vi "Perform Memory Polynomial.vi"(0 "RFmx Instrument Handle In":refnum<k21>, 1 "Selector String":string, 5 "RFSG Instrument Handle In":refnum<k15>, 7 "Reference Waveform":T2={"Name"="Wfm", "Data"=refnum, "Signal Bandwidth (Hz)"=0.0, "PAPR (dB)"=0.0, "Burst Length (s)"=0.0, "Sample Rate"=0.0, "Burst Start Locations"=[], "Burst Stop Locations"=[], "Idle Duration Present?"=FALSE, "Runtime Scaling"=0.0, "Script"=""} {"Runtime Scaling" format="%#_6p"; "Sample Rate" format="%#_6p"; "Burst Length (s)" format="%#_6p"; "PAPR (dB)" format="%.2f"; "Signal Bandwidth (Hz)" format="%#_6p"}, 9 "Memory Polynomial Configuration":T4={"Correction Type"=0, "Number of Iterations"=3, " Order"=3, " Depth"=2, "Lead Order"=2, "Lag Order"=2, "Lead Memory Depth"=2, "Lag Memory Depth"=2, "Maximum Lead"=2, "Maximum Lag"=2} {"Number of Iterations" min=1; "Correction Type" items=["Magnitude and Phase", "Magnitude Only", "Phase Only"]}, 11 "error in (no error)":errorcluster) -> (4 "RFmx Instrument Handle Out":refnum<k21> caption="Instrument Handle Out", 6 "RFSG Instrument Handle Out":refnum<k15>, 8 "Memory Polynomial Results":T1={"Predistorted Waveform"={"Name"="Wfm", "Data"=refnum, "Signal Bandwidth (Hz)"=0.0, "PAPR (dB)"=0.0, "Burst Length (s)"=0.0, "Sample Rate"=0.0, "Burst Start Locations"=[], "Burst Stop Locations"=[], "Idle Duration Present?"=FALSE, "Runtime Scaling"=0.0, "Script"=""}, "Polynomial"=[], "Power Results"={"Waveform Power Offset (dB)"=-1.0, "Waveform True PAPR (dB)"=0.0, "Training Power (dBm)"=0.0}} {"Power Results"."Training Power (dBm)" format="%.2f"; "Power Results"."Waveform True PAPR (dB)" format="%.2f"; "Power Results"."Waveform Power Offset (dB)" format="%.2f"; "Predistorted Waveform"."Runtime Scaling" format="%#_6p"; "Predistorted Waveform"."Sample Rate" format="%#_6p"; "Predistorted Waveform"."Burst Length (s)" format="%#_6p"; "Predistorted Waveform"."PAPR (dB)" format="%.2f"; "Predistorted Waveform"."Signal Bandwidth (Hz)" format="%#_6p"; "Polynomial" format="%.2f"}, 15 "error out":errorcluster)   [LabVIEW 2019, in "RFmxDPD.lvlib"]
doc: "Acquires the incoming signal, trains the DPD model, applies the memory polynomial to the reference waveform, and downloads the predistorted waveform to the generator. If generation is in progress when this function is called, generation will resume with the predistorted waveform."
uses:
  RFmxDPD.lvlib
  Common/Waveform.ctl
  Typedefs/Memory Polynomial Configuration.ctl
  Typedefs/Memory Polynomial Results.ctl
  Typedefs/Power Results.ctl
  <vilib>/RFmx/SpecAn/mx/RFmxSpecAn.llb/RFmxSpecAn DPD Fetch DPD Polynomial.vi
  SG/SG.lvlib
  Common/Common.lvlib
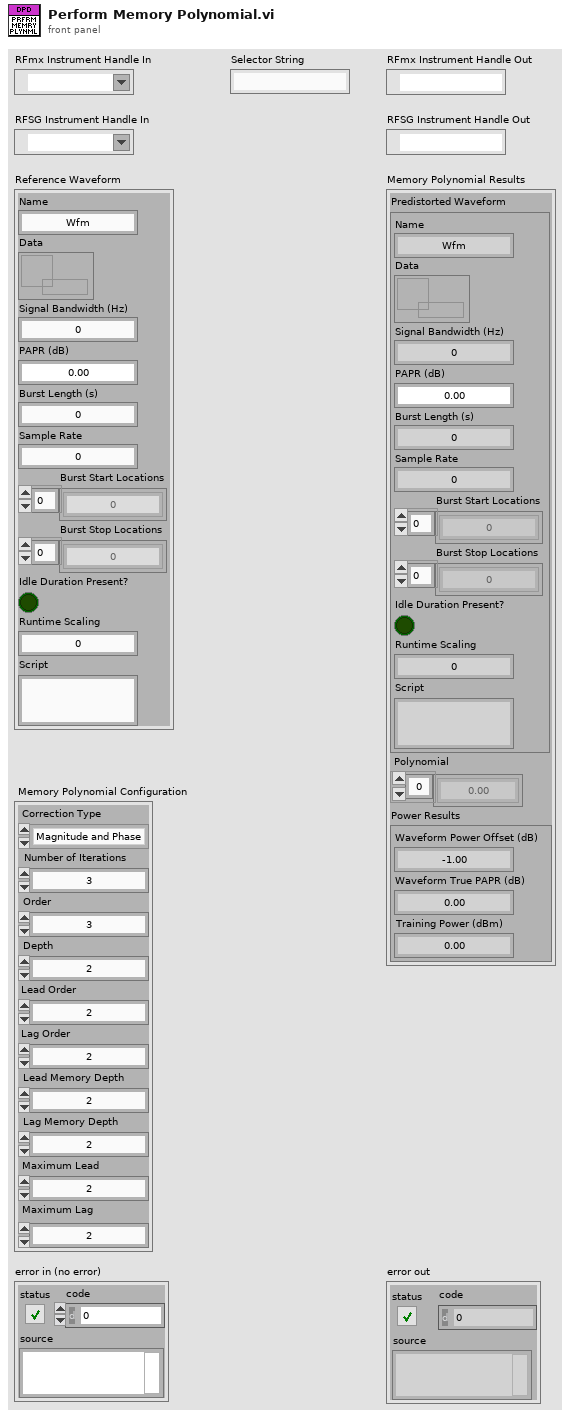
[diagram p1: front panel]
types:
  T1 = typedef "RFmxDPD.lvlib/Memory Polynomial Results.ctl" = cluster{"Predistorted Waveform":T2, "Polynomial":csg[], "Power Results":T3}
  T2 = typedef "Common.lvlib/Waveform.ctl" = cluster{"Name":string, "Data":refnum<data-value>, "Signal Bandwidth (Hz)":dbl, "PAPR (dB)":dbl, "Burst Length (s)":dbl, "Sample Rate":dbl, "Burst Start Locations":i32[], "Burst Stop Locations":i32[], "Idle Duration Present?":bool, "Runtime Scaling":dbl, "Script":string}
  T3 = typedef "RFmxDPD.lvlib/Power Results.ctl" = cluster{"Waveform Power Offset (dB)":dbl, "Waveform True PAPR (dB)":dbl, "Training Power (dBm)":dbl}
  T4 = typedef "RFmxDPD.lvlib/Memory Polynomial Configuration.ctl" = cluster{"Correction Type":i32, "Number of Iterations":i32, " Order":i32, " Depth":i32, "Lead Order":i32, "Lag Order":i32, "Lead Memory Depth":i32, "Lag Memory Depth":i32, "Maximum Lead":i32, "Maximum Lag":i32}
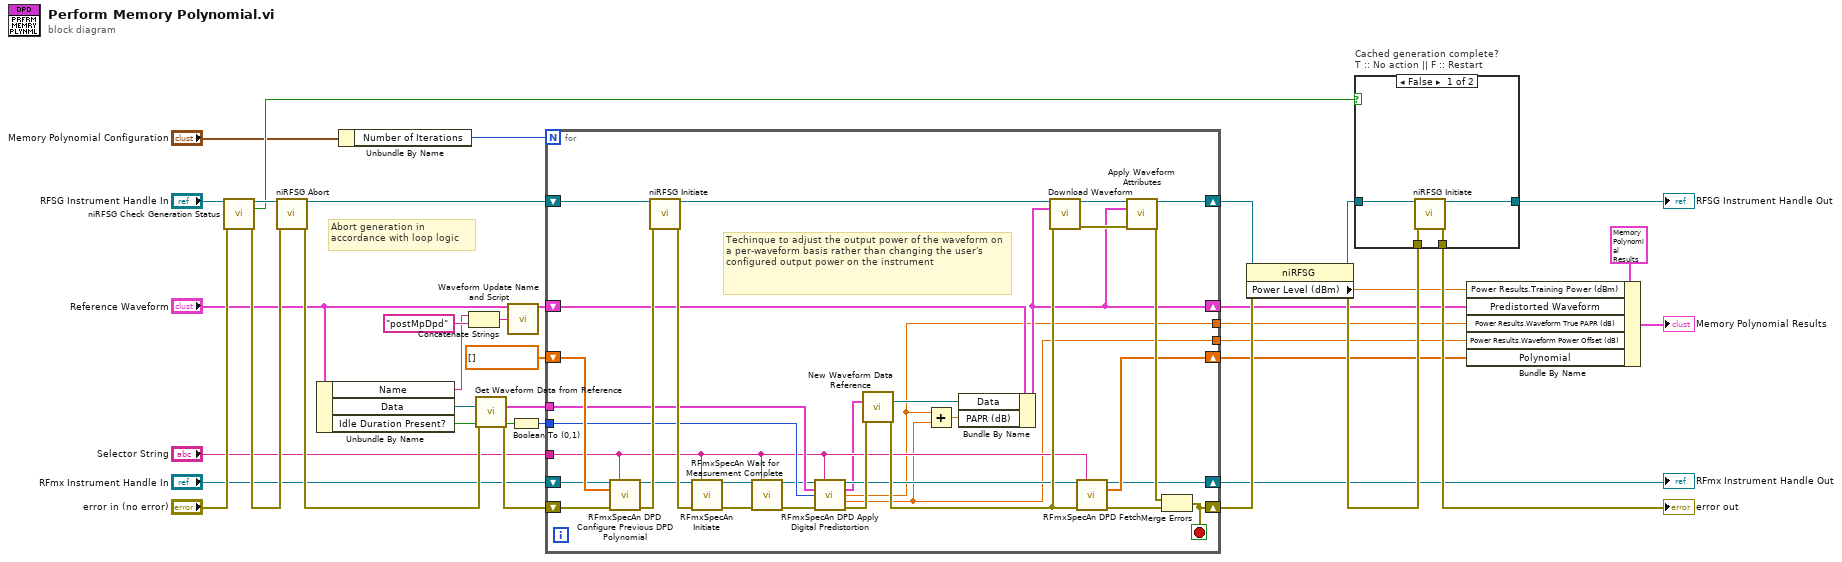
[diagram p0: block diagram]
diagram:
  # "Abort generation in\naccordance with loop logic"
  n1 = call <instrlib>:"niRFSG Check Generation Status.vi"("instrument handle"="RFSG Instrument Handle In", "error in"="error in (no error)") -> ("instrument handle out"=w23:refnum<k15>, "done?"=w21:bool, "error out"=w36:errorcluster)  [unwired: 11 in]
  n2 = call <instrlib>:"niRFSG Abort.vi"("instrument handle"=w23, "error in"=w36) -> ("instrument handle out"=w13:refnum<k15>, "error out"=w32:errorcluster)  [unwired: 12 in]
  n3 = Unbundle By Name("Reference Waveform") -> ("Name"=w2:string, "Data"=w19:refnum<data-value>, "Idle Duration Present?"=w18:bool)
  n4 = Unbundle By Name("Memory Polynomial Configuration") -> ("Number of Iterations"=w26:i32)
  n5 = Concatenate Strings(w2, "postMpDpd" ("string")) -> (w1:string)
  n6 = call "Get Waveform Data from Reference.vi"("Waveform Data Reference"=w19, "error in (no error)"=w32) -> ("Waveform Data"=w6:cluster{"t0":dbl, "dt":dbl, "y":csg[]}, "error out"=w31:errorcluster)  [unwired: 12 in]
  n7 = call "Waveform Update Name and Script.vi"("Waveform in"="Reference Waveform", "New Waveform Name"=w1) -> ("Waveform out"=w3:T2)  [unwired: 13 in]
  n8 = Boolean To (0,1)(Boolean=w18) -> (0, 1=w17:i16)
  n9 = for {
    N: w26 -> [_]
    shift-right: [w49] -> w10
    shift-left: "RFmx Instrument Handle In" -> [w55]
    shift-right: [w66] -> w34
    shift-left: w31 -> [w69]
    shift-right: [w54] -> w14
    shift-left: csg[] [] ("DPD Polynomial") -> [w57]
    tunnel: "Selector String" -> [w42]
    shift-right: [w47] -> w11
    shift-left: w13 -> [w46]
    shift-right: [w48] -> w25
    shift-left: w3 -> [w53]
    tunnel: w6 -> [w52]
    tunnel: w17 -> [w51]
    tunnel: [w40] -> w16
    tunnel: [w41] -> w15
    stop <- w66 stop-if-true
    # "Techinque to adjust the output power of the waveform on a per-waveform basis rather than changing the user's configured output power on the instrument"
    n10 = call <vilib>:"RFmxSpecAn DPD Configure Previous DPD Polynomial.vi"("Instrument Handle In"=w55, "Selector String"=w42, "Previous DPD Polynomial"=w57, "error in (no error)"=w69) -> ("Instrument Handle Out"=w56:refnum<k21>, "error out"=w65:errorcluster)  [unwired: 10 in]
    n11 = call <instrlib>:"niRFSG Initiate.vi"("instrument handle"=w46, "error in"=w65) -> ("instrument handle out"=w45:refnum<k15>, "error out"=w64:errorcluster)  [unwired: 12 in]
    n12 = call <vilib>:"RFmxSpecAn Initiate.vi"("Instrument Handle In"=w56, "Selector String"=w42, "error in (no error)"=w64) -> ("Instrument Handle Out"=w44:refnum<k21>, "error out"=w68:errorcluster)  [unwired: 10 in, 1 out]
    n13 = call <vilib>:"RFmxSpecAn Wait for Measurement Complete.vi"("Instrument Handle In"=w44, "Selector String"=w42, "error in (no error)"=w68) -> ("Instrument Handle Out"=w43:refnum<k21>, "error out"=w63:errorcluster)  [unwired: 11 in]
    n14 = call <vilib>:"RFmxSpecAn DPD Apply Digital Predistortion.vi"("Instrument Handle In"=w43, "Selector String"=w42, "Waveform In"=w52, "Idle Duration Present"=w51, "error in (no error)"=w63) -> ("Instrument Handle Out"=w50:refnum<k21>, "Waveform Out"=w37:cluster{"x0":dbl, "dx":dbl, "y":csg[]}, "PAPR (dB)"=w41:dbl, "Power Offset (dB)"=w40:dbl, "error out"=w61:errorcluster)  [unwired: 6 in]
    n15 = call "New Waveform Data Reference.vi"("Waveform Data"=w37, "error in (no error)"=w61) -> ("Waveform Data Reference"=w58:refnum<data-value>, "error out"=w59:errorcluster)  [unwired: 12 in]
    n16 = Add(x=w41, y=w40) -> (x+y=w39:dbl)
    n17 = Bundle By Name(cluster=w53, "Data"=w58, "PAPR (dB)"=w39) -> (w48:T2)
    n18 = call "Download Waveform.vi"("RFSG handle"=w45, "Waveform In"=w48, "error in (no error)"=w59) -> ("RFSG handle out"=w38:refnum<k15>, "error out"=w62:errorcluster)  [unwired: 11 in]
    n19 = call-poly <vilib>:"RFmxSpecAn DPD Fetch.vi"("Instrument Handle In"=w50, "Selector String"=w42, "error in (no error)"=w59) -> ("Instrument Handle Out"=w49:refnum<k21>, "DPD Polynomial"=w54:csg[], "error out"=w67:errorcluster)  [unwired: 10 in]
    n20 = call "Apply Waveform Attributes.vi"("RFSG Session In"=w38, "Waveform"=w48, "error in (no error)"=w62) -> ("RFSG Session Out"=w47:refnum<k15>, "error out"=w60:errorcluster)  [unwired: 11 in]
    n21 = Merge Errors(w60, w67) -> (w66:errorcluster)
  }
  "RFmx Instrument Handle Out" <- w10
  n22 = property class="niRFSG"(reference=w11, error in=w34) -> (reference out=w12:refnum<k15>, error out=w33:errorcluster, "Power Level (dBm)"=w9:dbl)
  n23 = case "Cached generation complete?\nT :: No action || F :: Restart" shown="False" w21 {
    tunnel: w12 -> [w71 w74]
    tunnel: [w70 w74] -> w22
    tunnel: w33 -> [w73 w75]
    tunnel: [w72 w75] -> w35
    frame False {
      n24 = call <instrlib>:"niRFSG Initiate.vi"("instrument handle"=w71, "error in"=w73) -> ("instrument handle out"=w70:refnum<k15>, "error out"=w72:errorcluster)  [unwired: 12 in]
    }
    frame True {
    }
  }
  "error out" <- w35
  "RFSG Instrument Handle Out" <- w22
  n25 = Bundle By Name(cluster=T1 {"Predistorted Waveform"={"Name"="Wfm", "Data"=refnum, "Signal Bandwidth (Hz)"=0.0, "PAPR (dB)"=0.0, "Burst Length (s)"=0.0, "Sample Rate"=0.0, "Burst Start Locations"=[], "Burst Stop Locations"=[], "Idle Duration Present?"=FALSE, "Runtime Scaling"=0.0, "Script"=""}, "Polynomial"=[], "Power Results"={"Waveform Power Offset (dB)"=-1.0, "Waveform True PAPR (dB)"=0.0, "Training Power (dBm)"=0.0}} ("Memory Polynomial Results"), "Power Results.Training Power (dBm)"=w9, "Predistorted Waveform"=w25, "Power Results.Waveform True PAPR (dB)"=w15, "Power Results.Waveform Power Offset (dB)"=w16, "Polynomial"=w14) -> (→"Memory Polynomial Results":T1)
